vi "Solenoid Globals.vi"() -> ()   [LabVIEW 2019]
panel:
  in  "Intake_Right_Extend":string="Intake_Right_Extend"
  in  "Hopper/Climb":string="Hopper/Climb"
  in  "Control_Panel":string="Control_Panel"
  in  "Intake_Left_Extend":string="Intake_Left_Extend"
  in  "Compressor":string="Compressor"
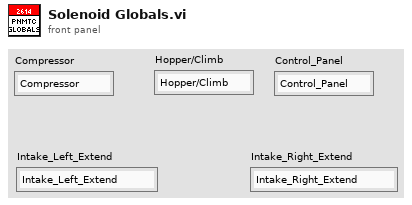
[diagram p1: front panel]
diagram:
